vi "HP34401A_CommandsGlobal.vi"() -> ()   [LabVIEW 2019, in "HP34401A.lvclass"]
uses:
  HP34401A.lvclass
panel:
  in  "HP34401A GPIB Setup":T1={"Instrument name"="HP34401A", "Command \"Reset\""="*RST", "Command \"Initialise\""="FUNC \"VOLT:DC\";VOLT:DC:RANG:AUTO 1; ", "Command \"Read Data\""=":READ?"}
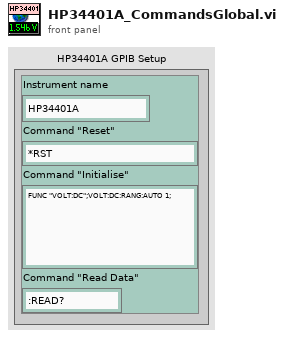
[diagram p1: front panel]
types:
  T1 = cluster{"Instrument name":string, "Command \"Reset\"":string, "Command \"Initialise\"":string, "Command \"Read Data\"":string}
diagram:
